vi "ReadSyringeConfiguration.vi"(0 "object in":refnum<class "CetoniPump.lvclass">, 5 "error in (no error)":errorcluster) -> (14 "object out":refnum<class "CetoniPump.lvclass">, 16 "COnfigured Syringes":T1(array[cluster]), 19 "error out":errorcluster)   [LabVIEW 2021, in "CetoniPump.lvclass"]
uses:
  CetoniPump.lvclass
  CetoniPump.lvclass/CetoniPump.ctl
  Users/olaja/AppData/Local/CETONI_SDK/lib/labview/labbCAN_Pump_API/labbCAN_Pump_API.lvlib
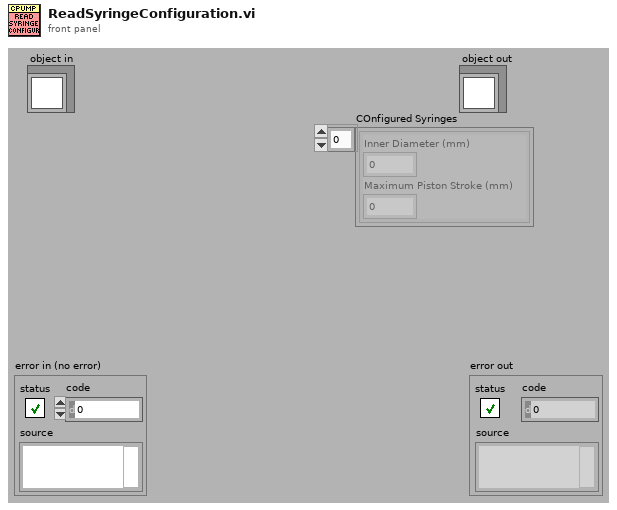
[diagram p1: front panel]
types:
  T1 = cluster{"Inner Diameter (mm)":dbl, "Maximum Piston Stroke (mm)":dbl}[]
  T2 = cluster{"Pump Handle":i64, "Pump Name":string, "Maximum Volume":dbl, "Maximum Flow Rate":dbl, "Flow Rate":dbl, "Target Level":dbl}[]
  T3 = cluster{"Inner Diameter (mm)":dbl, "Maximum Piston Stroke (mm)":dbl}
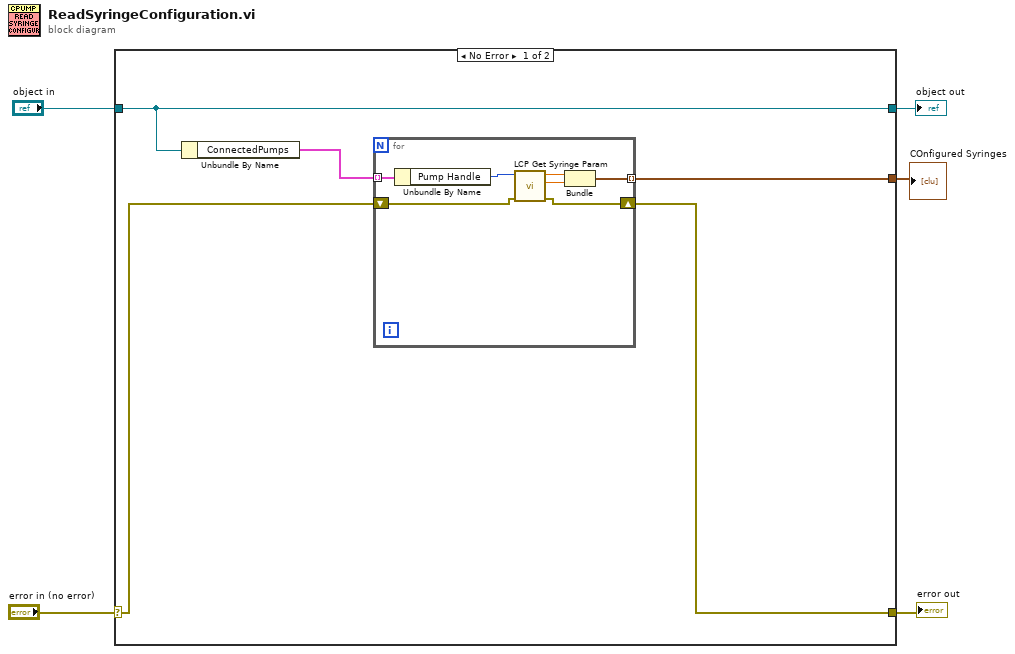
[diagram p0: block diagram]
diagram:
  n1 = case shown="No Error" "error in (no error)" {
    selector: "error in (no error)" -> [w8 w19]
    tunnel: [w7 w19] -> w4
    tunnel: [w10 w18] -> w2
    tunnel: "object in" -> [w10 w18]
    tunnel: [w6 _] -> w1
    frame No Error {
      n2 = Unbundle By Name(w10) -> ("ConnectedPumps"=w9:T2)
      n3 = for {
        tunnel: w9 -> [w17] mode=indexing
        shift-right: [w14] -> w7
        shift-left: w8 -> [w15]
        tunnel: [w11] -> w6 mode=indexing
        n4 = Unbundle By Name(w17) -> ("Pump Handle"=w16:i64)
        n5 = call "LCP Get Syringe Param.vi"("error in (no error)"=w15, "Pump Handle"=w16) -> ("error out"=w14:errorcluster, "Maximum Piston Stroke (mm)"=w13:dbl, "Inner Diameter (mm)"=w12:dbl)  [unwired: 7 in]
        n6 = Bundle("Inner Diameter (mm)"=w12, "Maximum Piston Stroke (mm)"=w13) -> (w11:T3)  [unwired: 1 in]
      }
    }
    frame Error {
    }
  }
  "error out" <- w4
  "object out" <- w2
  "COnfigured Syringes" <- w1
